vi "Packer. 1-I16 As U32.vi"(8 "Input Valid":bool=TRUE, 11 "Input data":cluster{"d0":i16, "d1":i16, "d2":i16, "d3":i16}) -> (0 "Output Valid":bool=TRUE, 3 "Output Data":u64)   [LabVIEW 2011]
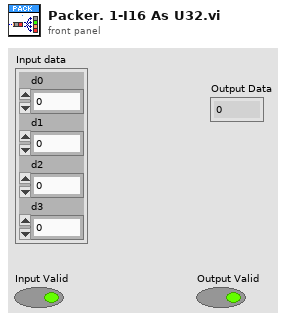
[diagram p1: front panel]
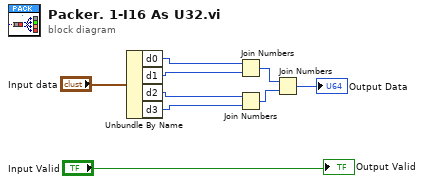
[diagram p0: block diagram]
diagram:
  n1 = Unbundle By Name("Input data") -> ("d0"=w7:i16, "d1"=w6:i16, "d2"=w5:i16, "d3"=w4:i16)
  n2 = Join Numbers(hi=w7, lo=w6) -> ((hi.lo)=w8:u32)
  n3 = Join Numbers(hi=w5, lo=w4) -> ((hi.lo)=w9:u32)
  n4 = Join Numbers(hi=w8, lo=w9) -> ((hi.lo)=→"Output Data":u64)
  "Output Valid" <- "Input Valid"
